vi "Get Control Terminals.vi"(8 "error in (no error)":errorcluster, 11 "VI in":refnum<vi>) -> (0 "error out":errorcluster, 2 "Controls":map{string, refnum<vi>}(c390), 3 "VI out":refnum<vi>)   [LabVIEW 2020, in "Responsive Mock Class Generator.lvclass"]
uses:
  Responsive Mock Class Generator.lvclass
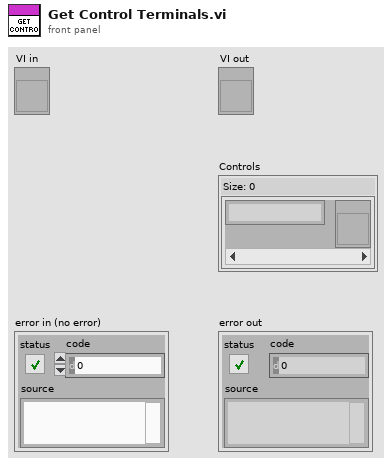
[diagram p1: front panel]
types:
  T1 = enum16{"Invalid Wire Rule", "Required", "Recommended", "Optional", "Dynamic Dispatch"}[]
  T2 = enum16{"Invalid Wire Rule", "Required", "Recommended", "Optional", "Dynamic Dispatch"}
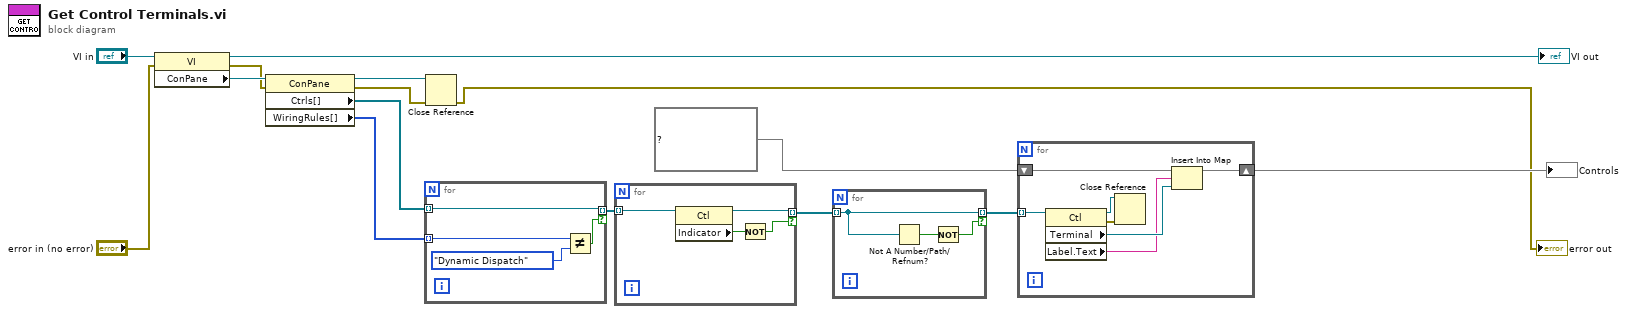
[diagram p0: block diagram]
diagram:
  n1 = property class="VI"(reference="VI in", error in="error in (no error)") -> (reference out=→"VI out":refnum<vi>, error out=w10:errorcluster, "ConPane"=w13:refnum<vi>)
  n2 = property class="ConPane"(reference=w13, error in=w10) -> (reference out=w11:refnum<vi>, error out=w12:errorcluster, "Ctrls[]"=w6:refnum<vi>[], "WiringRules[]"=w5:T1)
  n3 = for {
    tunnel: w6 -> [w17] mode=indexing
    tunnel: w5 -> [w19] mode=indexing
    tunnel: [w17] -> w4 mode=indexing if=w16
    n4 = Not Equal?(x=w19, y=T2."Dynamic Dispatch") -> (x != y?=w16:bool)
  }
  n5 = Close Reference(reference=w11, error in (no error)=w12) -> (error out=→"error out":errorcluster)
  n6 = for {
    tunnel: w4 -> [w23] mode=indexing
    tunnel: [w22] -> w2 mode=indexing if=w20
    n7 = property class="Ctl"(reference=w23) -> (reference out=w22:refnum<vi>, "Indicator"=w21:bool)  [unwired: 1 in, 1 out]
    n8 = Not(x=w21) -> (.not. x?=w20:bool)
  }
  n9 = for {
    tunnel: w2 -> [w26] mode=indexing
    tunnel: [w26] -> w1 mode=indexing if=w24
    n10 = Not A Number/Path/Refnum?(number/path/refnum=w26) -> (NaN/Path/Refnum?=w25:bool)
    n11 = Not(x=w25) -> (.not. x?=w24:bool)
  }
  n12 = for {
    shift-right: [w32] -> w7
    shift-left: map{string, refnum<vi>} {} ("map in") -> [w33]
    tunnel: w1 -> [w31] mode=indexing
    n13 = property class="Ctl"(reference=w31) -> (reference out=w28:refnum<vi>, error out=w29:errorcluster, "Terminal"=w30:refnum<vi>, "Label.Text"=w27:string)  [unwired: 1 in]
    n14 = Close Reference(reference=w28, error in (no error)=w29) -> ()  [unwired: 1 out]
    n15 = Insert Into Map(map in=w33, key=w27, value=w30) -> (map out=w32:map{string, refnum<vi>})  [unwired: 2 out]
  }
  "Controls" <- w7
